vi "catch.vi"(8 "error in (no error)":errorcluster, 9 "Position in":T1, 11 "catch position":cluster{i32, i32}) -> (0 "error out":errorcluster, 1 "Position out":T1)   [LabVIEW 2019]
uses:
  subVI/move/position cluster.ctl
  subVI/move control/move and align/move_cluster.ctl
  servo state.ctl
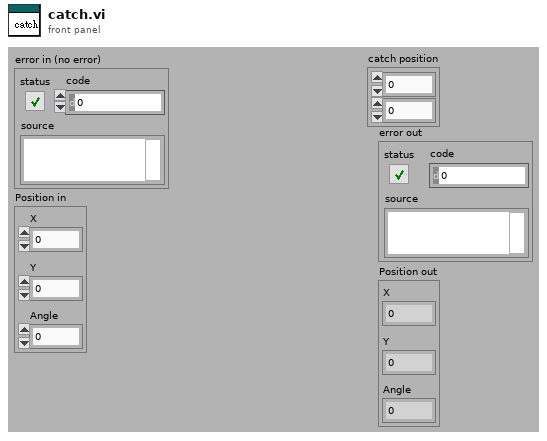
[diagram p1: front panel]
types:
  T1 = typedef "position cluster.ctl" = cluster{"X":dbl, "Y":dbl, "Angle":dbl}
  T2 = typedef "servo state.ctl" = enum16{"catch", "cam-1", "put", "side", "center", "side-2", "put-2"}
  T3 = typedef "move_cluster.ctl" = cluster{"X":dbl, "Y":dbl, "degree":dbl, "speed":dbl}
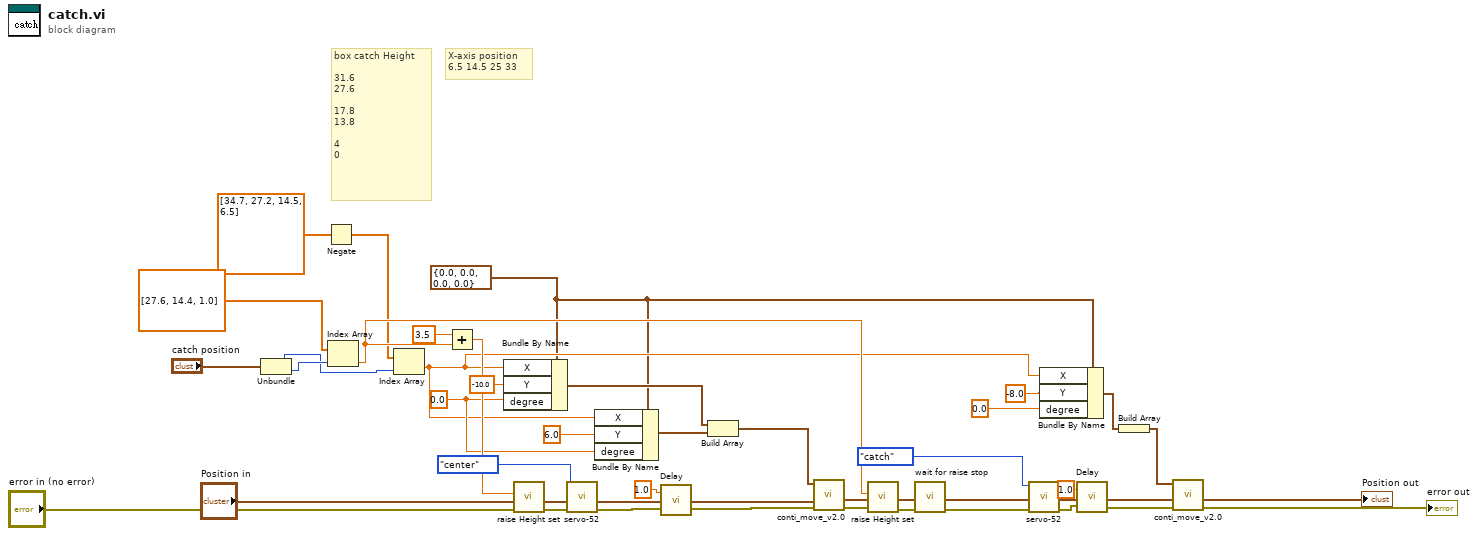
[diagram p0: block diagram]
diagram:
  w21 = 0.0 ("degree")
  w3 = T3 {"X"=0.0, "Y"=0.0, "degree"=0.0, "speed"=0.0} ("Cluster")
  # "X-axis position\n6.5 14.5 25 33"
  # "box catch Height\n\n31.6\n27.6\n\n17.8\n13.8\n\n4\n0"
  n1 = Unbundle("catch position") -> (w31:i32, w32:i32)
  n2 = Negate(x=dbl[] [34.7, 27.2, 14.5, 6.5]) -> (-x=w15:dbl[])
  n3 = Index Array(array=dbl[] [27.6, 14.4, 1.0], index=w32) -> (element=w19:dbl)
  n4 = Index Array(array=w15, index=w31) -> (element=w11:dbl)
  n5 = Add(x=3.5, y=w19) -> (x+y=w34:dbl)
  n6 = Bundle By Name(cluster=w3, "X"=w11, "Y"=-10.0, "degree"=w21) -> (w27:T3)
  n7 = call "raise Height set.vi"("error in (no error)"="error in (no error)", "Height_cm"=w34) -> ("error out"=w30:errorcluster)  [unwired: 9 in]
  n8 = call "servo-52.vi"("error in (no error)"=w30, "Enum"=servo_state."center") -> ("error out"=w24:errorcluster)  [unwired: 9 in]
  n9 = Bundle By Name(cluster=w3, "X"=w11, "Y"=6.0, "degree"=w21) -> (w26:T3)
  n10 = call "Delay.vi"("error in (no error)"=w24, "Delay Time (s)"=1.0) -> ("error out"=w22:errorcluster)  [unwired: 1 in]
  n11 = Build Array(w27, w26) -> (w25:T3[])
  n12 = call "conti_move_v2.0.vi"("error in (no error)"=w22, "Position"="Position in", "route"=w25) -> ("error out"=w20:errorcluster, "Position out"=w12:T1)  [unwired: 7 in]
  n13 = call "raise Height set.vi"("error in (no error)"=w20, "Height_cm"=w19) -> ("error out"=w17:errorcluster)  [unwired: 9 in]
  n14 = call "wait for raise stop.vi"("Error In"=w17) -> ("Error Out"=w16:errorcluster)  [unwired: 10 in]
  n15 = call "servo-52.vi"("error in (no error)"=w16, "Enum"=servo_state."catch") -> ("error out"=w14:errorcluster)  [unwired: 9 in]
  n16 = Bundle By Name(cluster=w3, "X"=w11, "Y"=-8.0, "degree"=0.0) -> (w4:T3)
  n17 = call "Delay.vi"("error in (no error)"=w14, "Delay Time (s)"=1.0) -> ("error out"=w13:errorcluster)  [unwired: 1 in]
  n18 = Build Array(w4) -> (w8:T3[])
  n19 = call "conti_move_v2.0.vi"("error in (no error)"=w13, "Position"=w12, "route"=w8) -> ("error out"=→"error out":errorcluster, "Position out"=→"Position out":T1)  [unwired: 7 in]
